vi "Clean Facade.vi"(8 "error in (no error)":errorcluster, 11 "SMOFacade in":refnum<class "SMOFacade.lvclass">) -> (0 "error out":errorcluster)   [LabVIEW 2013, in "SMOFacade.lvlib" / "SMOFacade.lvclass"]
uses:
  SMOFacade.lvclass
  SMOFacade.lvclass/SMOFacade.ctl
  Registry/SMO_API--Cluster.ctl
  Terminal/Terminal.lvclass
  Registry/Registry-SMO.lvclass
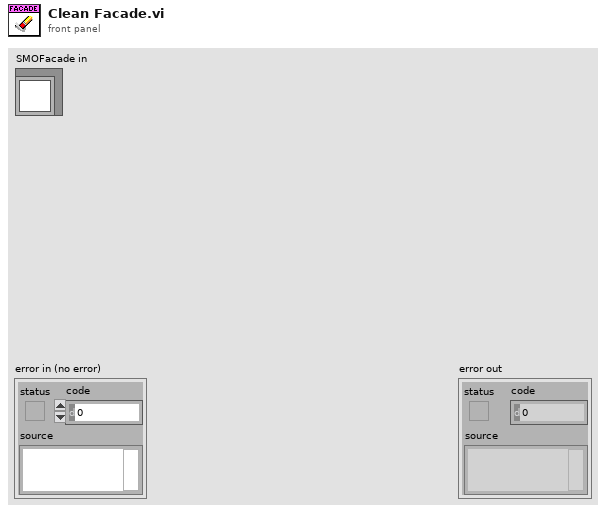
[diagram p1: front panel]
types:
  T1 = typedef "Registry-SMO.lvclass/SMO_API--Cluster.ctl" = cluster{"Method Name":string, "Full Method Name":string, "SMO Input":refnum<class "Terminal.lvclass">, "SMO Output":refnum<class "Terminal.lvclass">, "Inputs":refnum<class "Terminal.lvclass">[], "Outputs":refnum<class "Terminal.lvclass">[], "Error Output":refnum<class "Terminal.lvclass">, "vi reference":refnum<vi>}
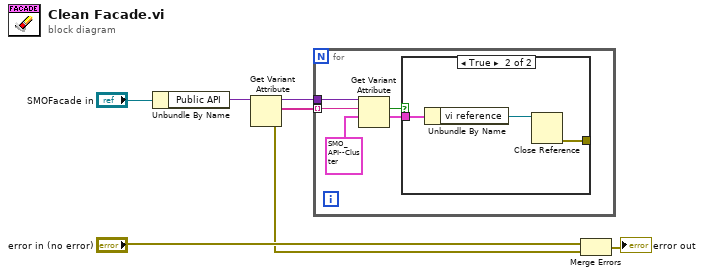
[diagram p0: block diagram]
diagram:
  n1 = Unbundle By Name("SMOFacade in") -> ("Public API"=w7:variant)
  n2 = Get Variant Attribute(Variant=w7) -> (duplicate Variant=w5:variant, names=w4:string[], error out=w2:errorcluster)  [unwired: 3 in, 1 out]
  n3 = for {
    tunnel: w5 -> [w12]
    tunnel: w4 -> [w11] mode=indexing
    n4 = Get Variant Attribute(Variant=w12, name=w11, default value (empty Variant)=T1 {"Method Name"="", "Full Method Name"="", "SMO Input"=refnum, "SMO Output"=refnum, "Inputs"=[], "Outputs"=[], "Error Output"=refnum, "vi reference"=refnum} ("API")) -> (found=w9:bool, value=w8:T1)  [unwired: 1 in, 2 out]
    n5 = case shown="True" w9 {
      tunnel: w8 -> [_ w15]
      tunnel: [_ w13] -> _
      frame False {
      }
      frame True {
        n6 = Unbundle By Name(w15) -> ("vi reference"=w14:refnum<vi>)
        n7 = Close Reference(reference=w14) -> (error out=w13:errorcluster)  [unwired: 1 in]
      }
    }
  }
  n8 = Merge Errors("error in (no error)", w2) -> (→"error out":errorcluster)
